vi "Query Limits and Protections.vi"(8 "error in (no error)":errorcluster, 11 "N5745A in":refnum<class "5745A.lvclass">) -> (0 "error out":errorcluster, 2 "Limits and Protections":T1 {"Voltage Limit" format="%.3f"; "UVL" format="%.3f"; "OVP" format="%.3f"; "Current Limit" format="%.3f"}, 3 "N5745A out":refnum<class "5745A.lvclass">)   [LabVIEW 2018, in "5745A.lvlib" / "5745A.lvclass"]
doc: "This method is used for querying the limits and protection setting on the N5745A Power Supply:\nVoltage Limit\nCurrent Limit\nOver Voltage Protection (OVL)\nUnder Voltage Limit (UVL)\nOver Current Protection (OCP)"
uses:
  5745A.lvclass
  Custom Controls/Limits and Protections.ctl
  builds/Power_Supply.lvlibp/Power Supply.lvclass
  C:/Users/Ron.Dexter.LUMINARTECH/Desktop/builds/Power_Supply.lvlibp/Power Supply.lvclass
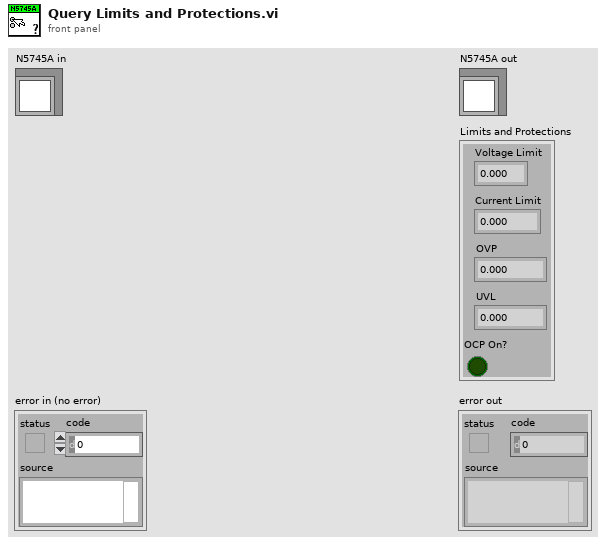
[diagram p1: front panel]
types:
  T1 = typedef "5745A.lvlib/5745A.lvclass/Limits and Protections.ctl" = cluster{"OCP On?":bool, "Current Limit":dbl, "OVP":dbl, "UVL":dbl, "Voltage Limit":dbl}
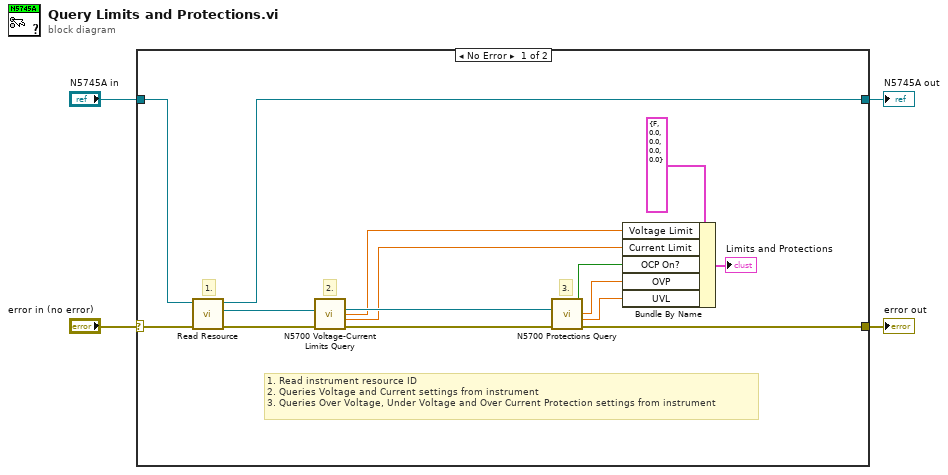
[diagram p0: block diagram]
diagram:
  n1 = case shown="No Error" "error in (no error)" {
    selector: "error in (no error)" -> [w11 w21]
    tunnel: [w7 w21] -> w3
    tunnel: [w5 w20] -> w1
    tunnel: "N5745A in" -> [w6 w20]
    frame No Error {
      # "1. Read instrument resource ID\n2. Queries Voltage and Current settings from instrument\n3. Queries Over Voltage, Under Voltage and Over Current Protection settings from instrument"
      # "3."
      # "2."
      # "1."
      n2 = call "Read Resource.vi"("error in"=w11, "Power Supply in"=w6) -> ("error out"=w8:errorcluster, "Resource"=w9:refnum<visa-resource-name>, "Power Supply out"=w5:refnum<class "5745A.lvclass">)  [unwired: 7 in]
      n3 = call <instrlib>:"N5700 Voltage-Current Limits Query.vi"("error"=w8, "VISA"=w9) -> ("error out"=w19:errorcluster, "Current Limit?"=w14:dbl, "Voltage Limit?"=w15:dbl, "VISA out"=w18:refnum<visa-resource-name>)  [unwired: 3 in]
      n4 = call <instrlib>:"N5700 Protections Query.vi"("error"=w19, "VISA"=w18) -> ("error out"=w7:errorcluster, "UVL"=w12:dbl, "OVP"=w13:dbl, "OCP"=w16:bool)  [unwired: 3 in, 1 out]
      n5 = Bundle By Name(cluster=T1 {"OCP On?"=FALSE, "Current Limit"=0.0, "OVP"=0.0, "UVL"=0.0, "Voltage Limit"=0.0} ("Limits and Protections"), "Voltage Limit"=w15, "Current Limit"=w14, "OCP On?"=w16, "OVP"=w13, "UVL"=w12) -> (→"Limits and Protections":T1)
    }
    frame Error {
    }
  }
  "error out" <- w3
  "N5745A out" <- w1
